vi "get_js_gonghao.vi"(8 "lc_num":string, 11 "juese":string) -> (0 "error":errorcluster caption="error out 4", 2 "jsren":string)   [LabVIEW 2017, in "Lib_code.lvlib"]
uses:
  Lib_code.lvlib
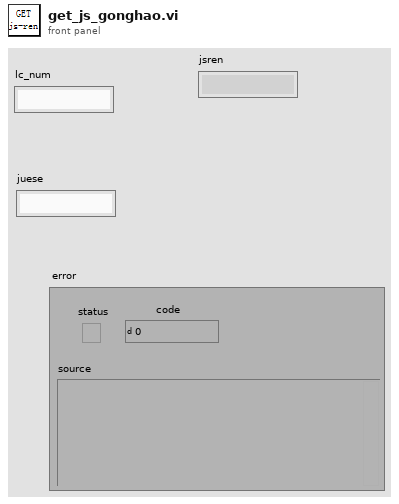
[diagram p1: front panel]
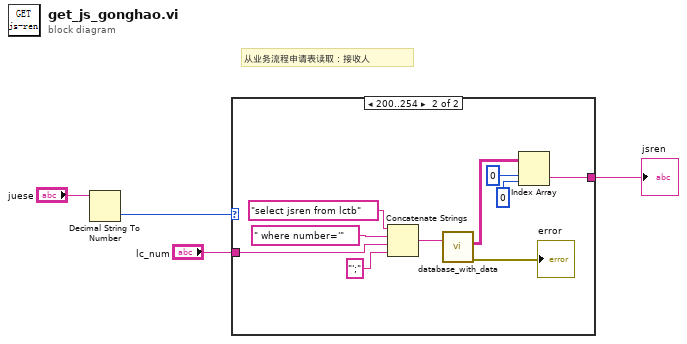
[diagram p0: block diagram]
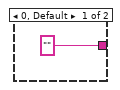
[diagram p2: hidden frame]
diagram:
  # "从业务流程申请表读取：接收人"
  n1 = Decimal String To Number(string="juese") -> (number=w2:i32)  [unwired: 2 in, 1 out]
  n2 = case shown="200..254" w2 {
    tunnel: "lc_num" -> [_ w15]
    tunnel: ["" ("String") w14] -> w3
    frame 0, Default {
    }
    frame 200..254 {
      n3 = Concatenate Strings("select jsren from lctb" ("Command Text"), " where number='" ("Command Text"), w15, "';" ("字符串")) -> (w8:string)
      n4 = call "database_with_data.vi"("input"=w8) -> ("error"=→"error":errorcluster, "Data"=w7:string[][])  [unwired: 9 in]
      n5 = Index Array(array=w7, index (row)=0 ("索引 (行)"), index (col)=0 ("禁用的索引 (列)")) -> (element=w14:string)
    }
  }
  "jsren" <- w3
